vi "Save_pupil_param.vi"(10 "Array":T1(array[cluster]), 11 "path":path) -> (0 "error out":errorcluster)   [LabVIEW 2018]
uses:
  <vilib>/Utility/file.llb/Write Delimited Spreadsheet (string).vi
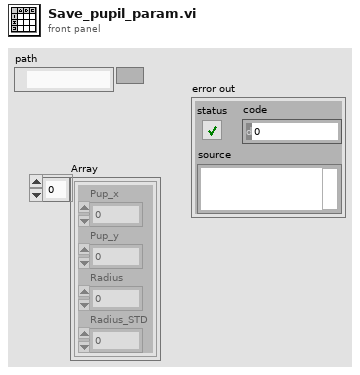
[diagram p1: front panel]
types:
  T1 = cluster{"Pup_x":i16, "Pup_y":i16, "Radius":i16, "Radius_STD":i16}[]
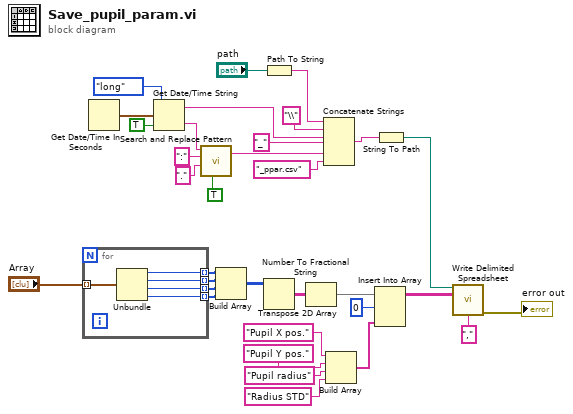
[diagram p0: block diagram]
diagram:
  n1 = for {
    tunnel: "Array" -> [w38] mode=indexing
    tunnel: [w37] -> w19 mode=indexing
    tunnel: [w36] -> w20 mode=indexing
    tunnel: [w35] -> w21 mode=indexing
    tunnel: [w34] -> w22 mode=indexing
    n2 = Unbundle(w38) -> ("Pup_x"=w37:i16, "Pup_y"=w36:i16, "Radius"=w35:i16, "Radius_STD"=w34:i16)
  }
  n3 = Get Date/Time In Seconds() -> (seconds since 1Jan1904=w3:timestamp)
  n4 = Get Date/Time String(date format (0)=enum16{"short", "long", "abbreviated"}."long", seconds (now)=w3, want seconds? (F)=TRUE) -> (date string=w6:string, time string=w15:string)
  n5 = call <vilib>:"Search and Replace Pattern.vi"("string"=w15, "regular expression (\"\")"=":" ("regular expression (\"\")"), "replace string (\"\")"="." ("replace string (\"\")"), "replace all? (F)"=TRUE) -> ("result string"=w14:string)  [unwired: 1 in, 1 out]
  n6 = Build Array(w19, w20, w21, w22) -> (w23:i16[][])
  n7 = Path To String(path="path") -> (string=w10:string)
  n8 = Number To Fractional String(number=w23) -> (F-format string=w31:string[][])  [unwired: 3 in]
  n9 = Transpose 2D Array(2D array=w31) -> (transposed array=w32:string[][])
  n10 = Concatenate Strings(w10, "\\" ("string"), w6, "_", w14, "_ppar.csv" ("string")) -> (w9:string)
  n11 = Build Array("Pupil X pos." ("string"), "Pupil Y pos." ("string"), "Pupil radius" ("string"), "Radius STD" ("string")) -> (w25:string[])
  n12 = Insert Into Array(array=w32, index (row)=0, new element=w25) -> (w33:string[][])  [unwired: 1 in]
  n13 = String To Path(string=w9) -> (path=w17:path)
  n14 = call-poly <vilib>:"Write Delimited Spreadsheet.vi"("file path (dialog if empty)"=w17, "2D data"=w33, "delimiter (\\t)"="," ("delimiter (\\t)")) -> ("error out"=→"error out":errorcluster)  [unwired: 11 in, 1 out]
